vi "TAT_Start.vi"(8 "error In":errorcluster) -> (0 "error out":errorcluster)   [LabVIEW 2017]
uses:
  <vilib>/Utility/error.llb/DialogType.ctl
  Controls/Ass. Loop Control.ctl
  <vilib>/addons/database/Connection.llb/Conn ObjectReference.ctl
  2ffc4e95-467e-4723-8c12-a792954531b5.vi
  8539105e-fe5f-4c29-a376-e00596b22cdb.vi
  <vilib>/addons/database/Connection.llb/DB Tools Open Connec (Path).vi
  Global/Global 1.vi
  <vilib>/Instr/_visa.llb/VISA Configure Serial Port (Instr).vi
  <vilib>/addons/database/NI_Database_API.lvlib
  <vilib>/Utility/config.llb/NI_LVConfig.lvlib
panel:
  out "PREVIOUS BARCODE":string
  out "PACKAGED QUANTITY":string
  out "SCANNED QUANTITY":string
  out "PACKAGE STICKER":string
  out "PRN to Print":string
  out "CYCLE RESULT:-":bool caption="LEAK RESULT:-"
  out "CYCLE STATUS STATION 2":string caption="CYCLE STATUS 2:-"
  out "SERIAL NO.:- 2":dbl
  out "PY1B-D-EX:-":bool caption="LEAK RESULT:-"
  out "PYIB-MD-EX:-":bool caption="LEAK RESULT:-"
  out "RBC-M-H:-":bool caption="LEAK RESULT:-"
  out "PY1B-D:-":bool caption="LEAK RESULT:-"
  out "PYIB-MD:-":bool caption="LEAK RESULT:-"
  out "HOSE:-":bool caption="LEAK RESULT:-"
  out "DUAL:-":bool caption="LEAK RESULT:-"
  out "RBC-M-EX:-":bool caption="LEAK RESULT:-"
  out "CAP SEAL:-":bool caption="LEAK RESULT:-"
  in  "Model Selection:-":string(combo)
  out "CYCLE TIME:-":u32
  out "BARCODE STATION 2":string caption="QR CODE :-"
  out "CYCLE START:-":bool caption="LEAK RESULT:-"
  out "PREVIOUS BARCODE":string[](array[string])
  out "scanned":string
  out "Scanned Qty  2":string
  out "PROJECT :-":string
  out "PACKAGE Qty":string
  out "TORISHI CODE:-":string
  out "PART No.:-":string
  out "PLC STATUS:-":bool
  in  "Stop":bool
  out "QR STATION 1":string caption="QR CODE:-"
  out "RESULT STATION 1":bool caption="FINAL RESULT:-"
  out "USER:-":string
  out "PART NAME :-":string
  in  "ASS-Alarms":bool
  out "CYCLE STATUS STATION 1":string caption="CYCLE STATUS 1:-"
  out "DATE/TIME":string
  # "KAPSE SONS ROBOTICS\n& AUTOMATION"
  # "MODEL SELECTION:-"
  # "Nm"
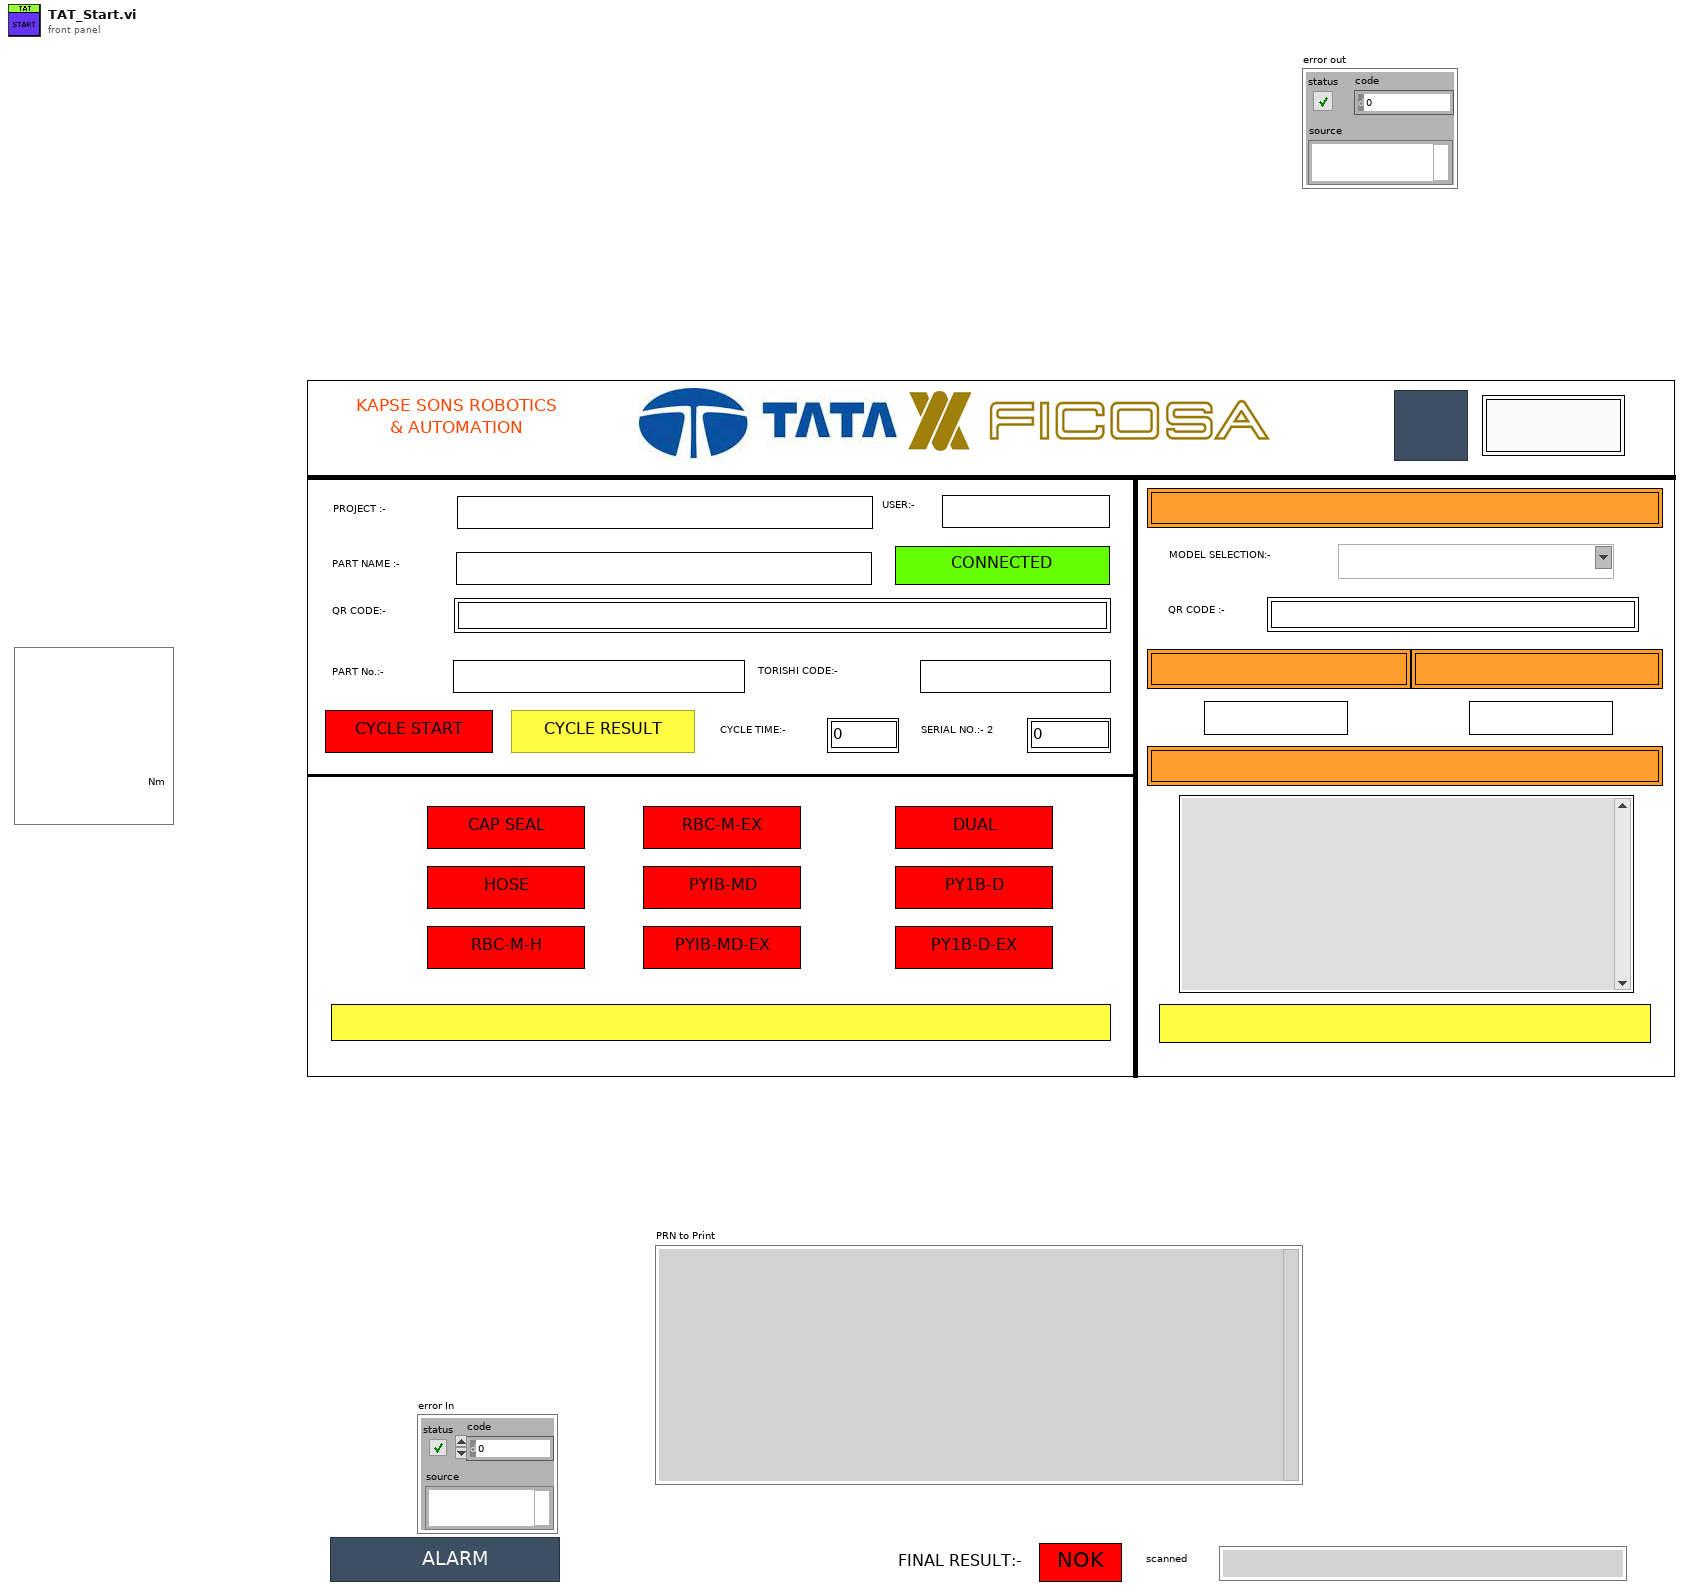
[diagram p1: front panel]
types:
  T1 = typedef "NI_Database_API.lvlib/Conn ObjectReference.ctl" = refnum<k1>
  T2 = cluster{"Varient number":u16, "Part name":string, "connection reference":T1, "Batch_Size":u16, "PART_NO":string, "TORISHI_CODE":string, "scanner com":refnum<visa-resource-name>, "Part Name List":string[], "Varient path":path, "Current Varient path":path, "Communication path":path, "Package path":path, "Part PRN path":path, "Station2 printer IP":string, "Station1 printer IP":string, "Current Serial Number":string, "Station1_QR":string, "Serial_Number":path, "PRIVIOUS code":string[], "Barcode station 2 to log Dn":string, "Barcode station 2 to log Up":string}
  T3 = cluster{"Varient number":u16, "Part name":string, "Barcode":string, "connection reference":T1, "Batch_Size":u16, "PART_NO":string, "TORISHI_CODE":string, "scanner com":refnum<visa-resource-name>, "Part Name List":string[], "Varient path":path, "Current Varient path":path, "Communication path":path, "Package path":path, "Part PRN path":path, "Station2 printer IP":string, "Station1 printer IP":string, "Current Serial Number":string, "Station1_QR":string, "Serial_Number":path, "PRIVIOUS code":string[], "Barcode station 2 to log":string}
  T4 = typedef "Ass. Loop Control.ctl" = enum16{"Package_Qty_Count", "GENERATE_QR_PRNT", "Cluster_update", "Waiting_for_scan", "barcode CHECK", "Int", "SaveReport ", "Barcode Print", "Start Cycle", "Wait", "Cycle End", "Stop"}
  T5 = typedef "DialogType.ctl" = u16
  T6 = enum32{"invalid app kind", "Development System", "Run Time System", "Student Edition", "Embedded LabVIEW", "Evaluation", "Custom"}
  T7 = typedef "NI_LVConfig.lvlib/Config Data RefNum.ctl" = refnum<k1>
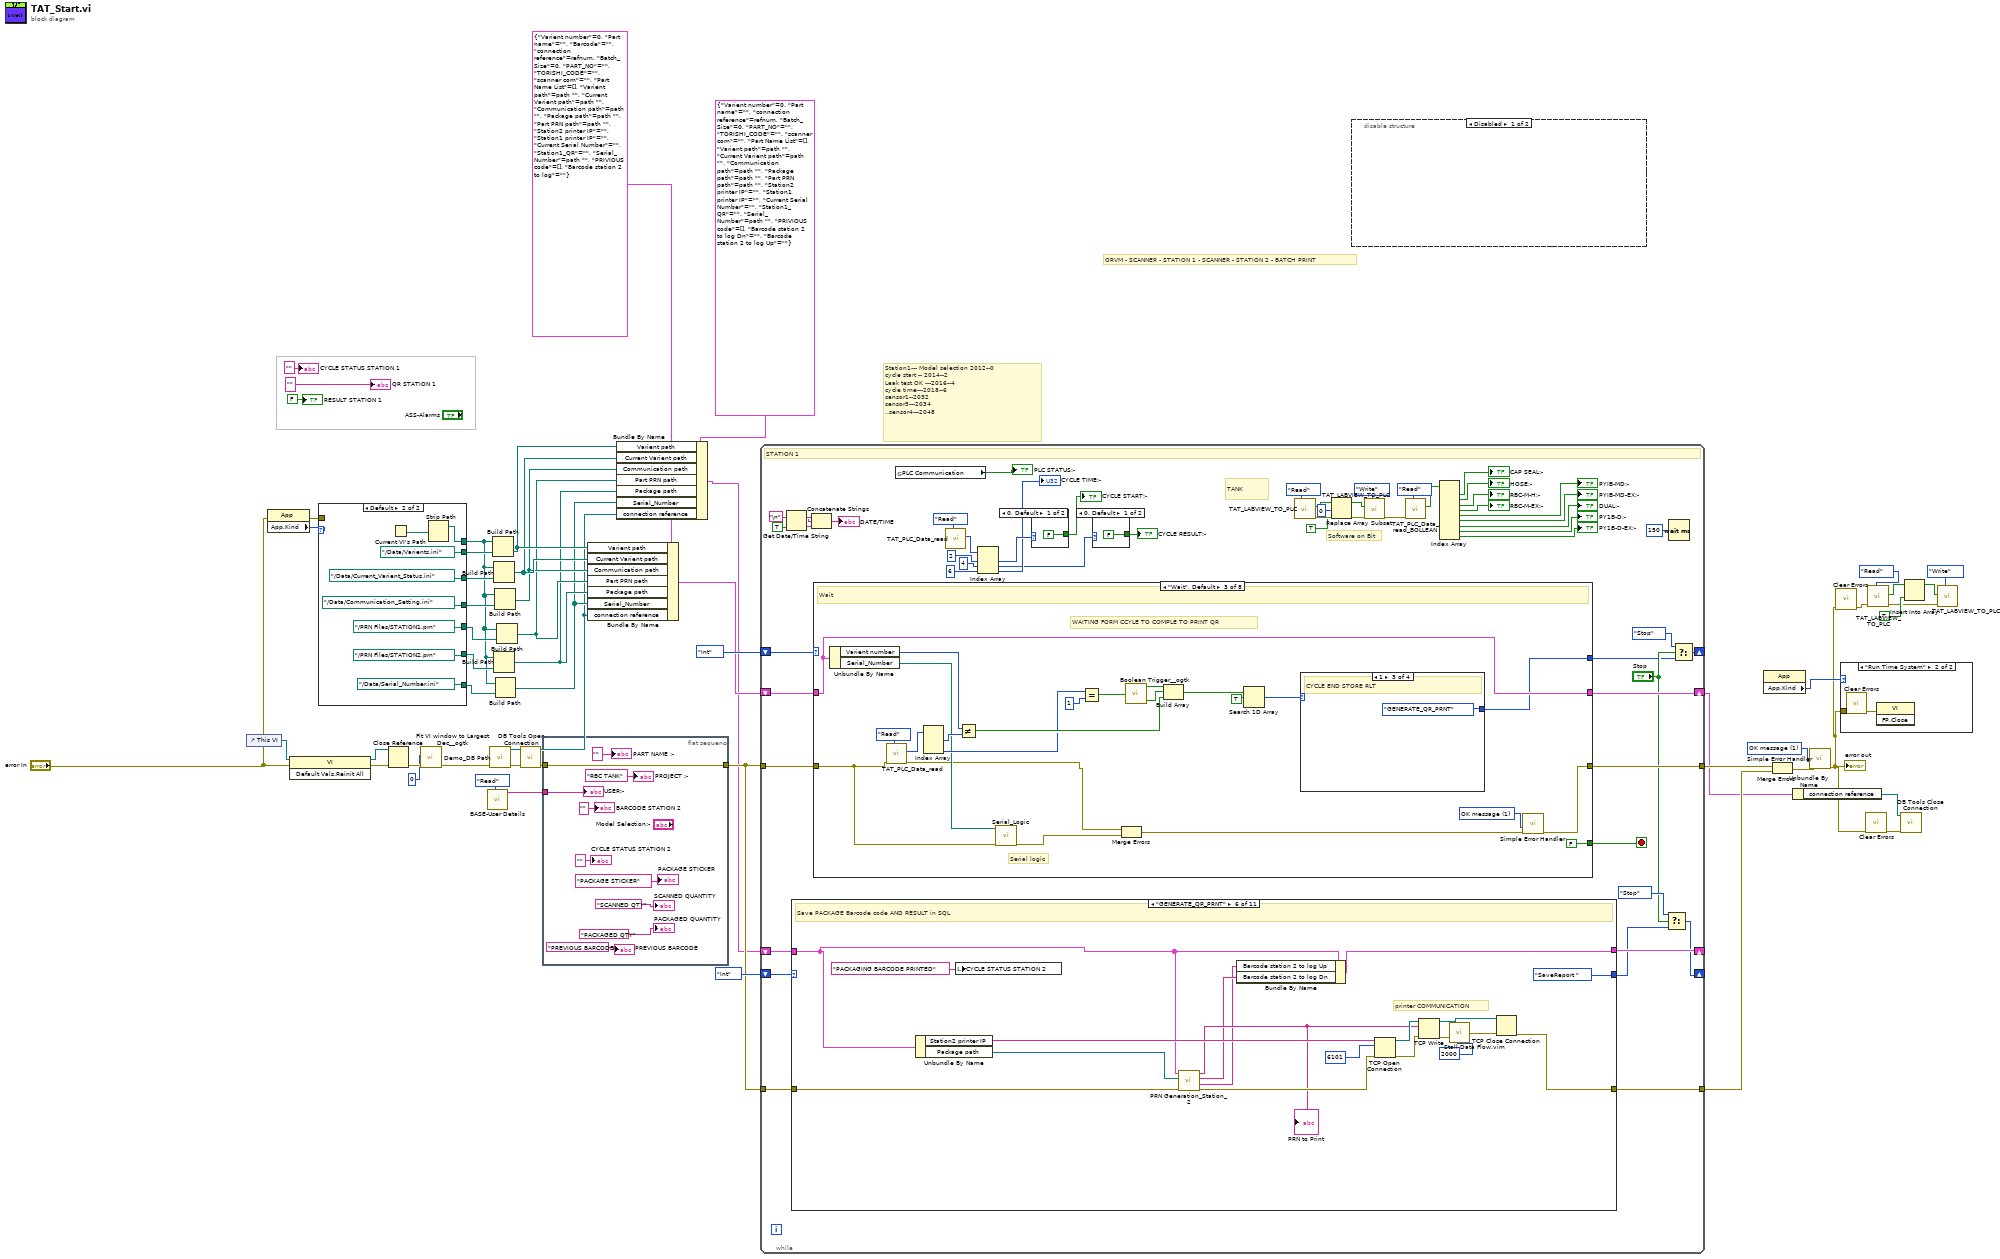
[diagram p0: block diagram]
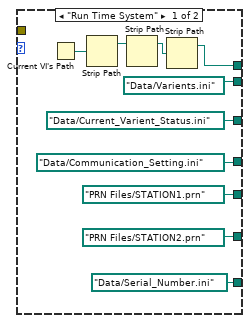
[diagram p2: hidden frame]
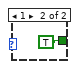
[diagram p5: hidden frame]
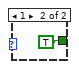
[diagram p6: hidden frame]
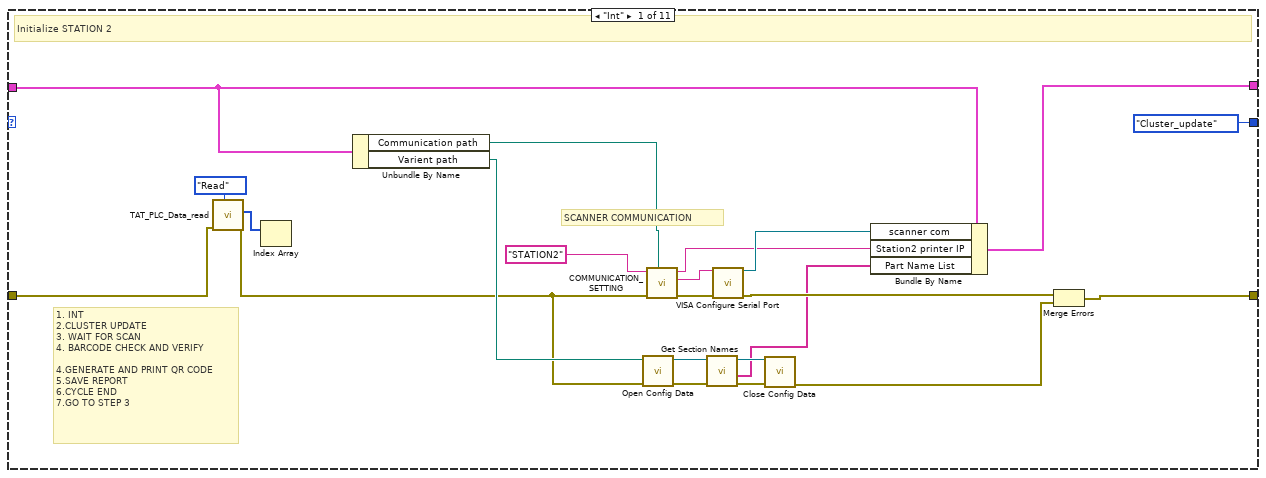
[diagram p7: hidden frame]
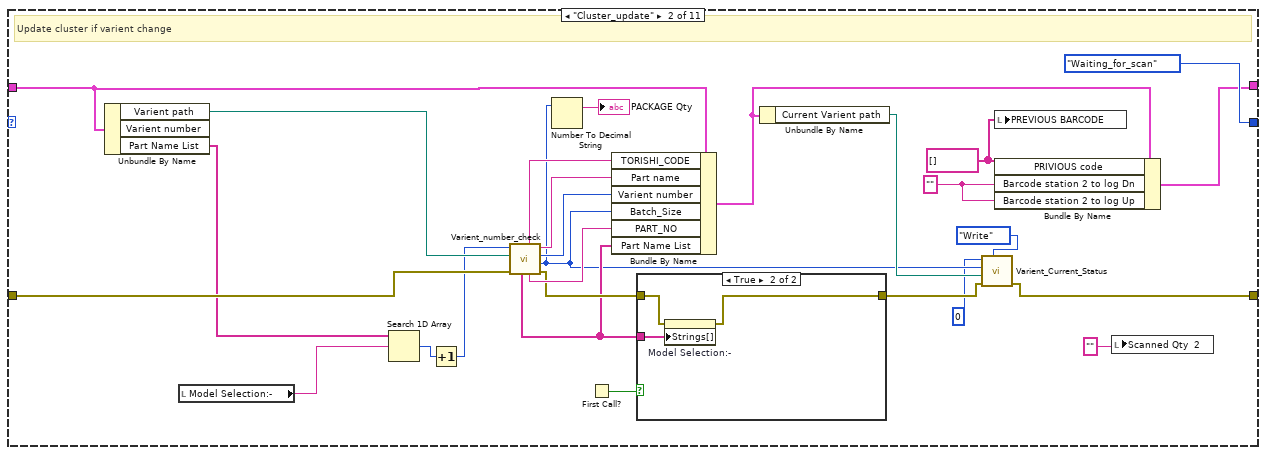
[diagram p8: hidden frame]
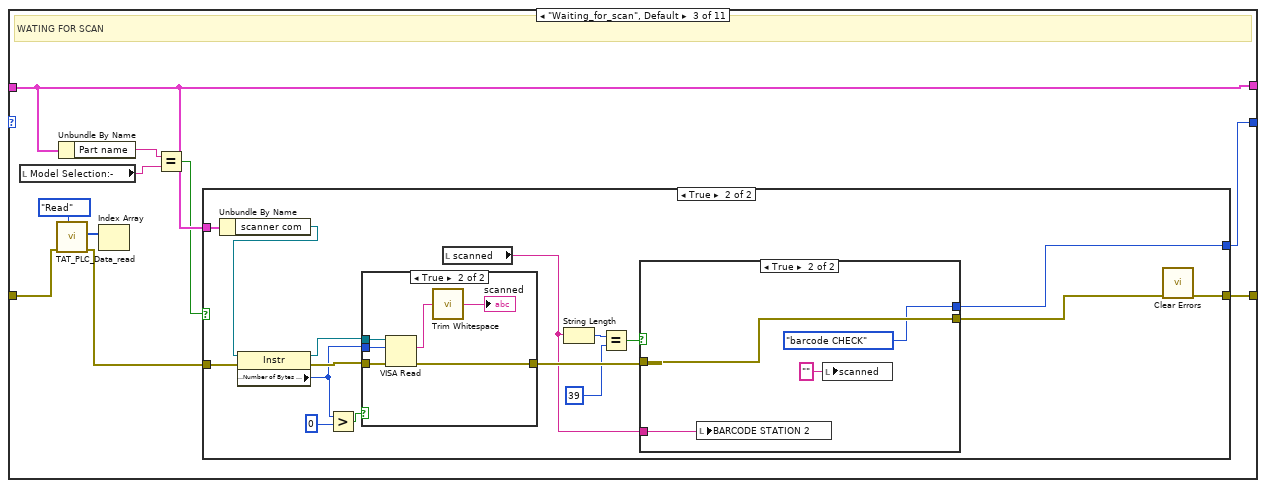
[diagram p10: hidden frame]
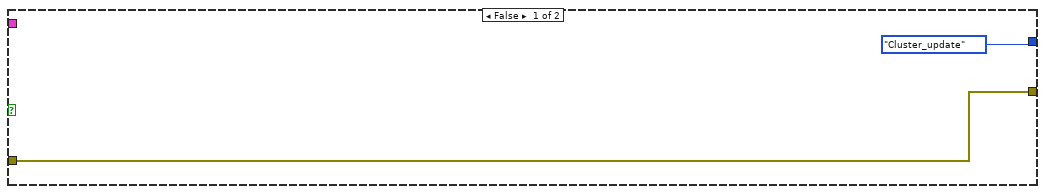
[diagram p11: hidden frame]
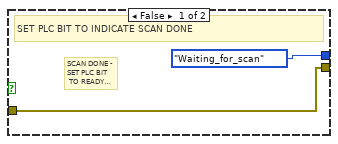
[diagram p13: hidden frame]
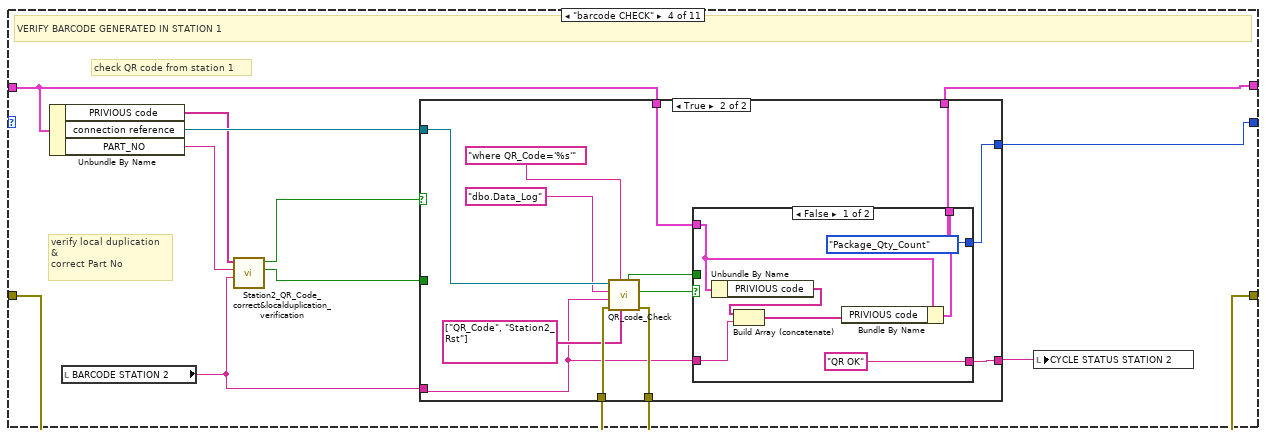
[diagram p14: hidden frame]
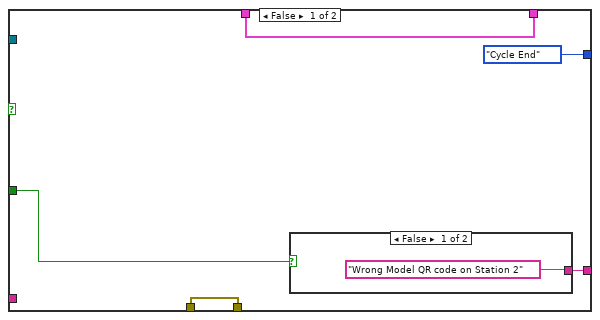
[diagram p15: hidden frame]
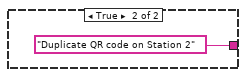
[diagram p16: hidden frame]
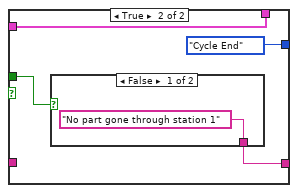
[diagram p17: hidden frame]
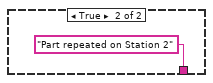
[diagram p18: hidden frame]
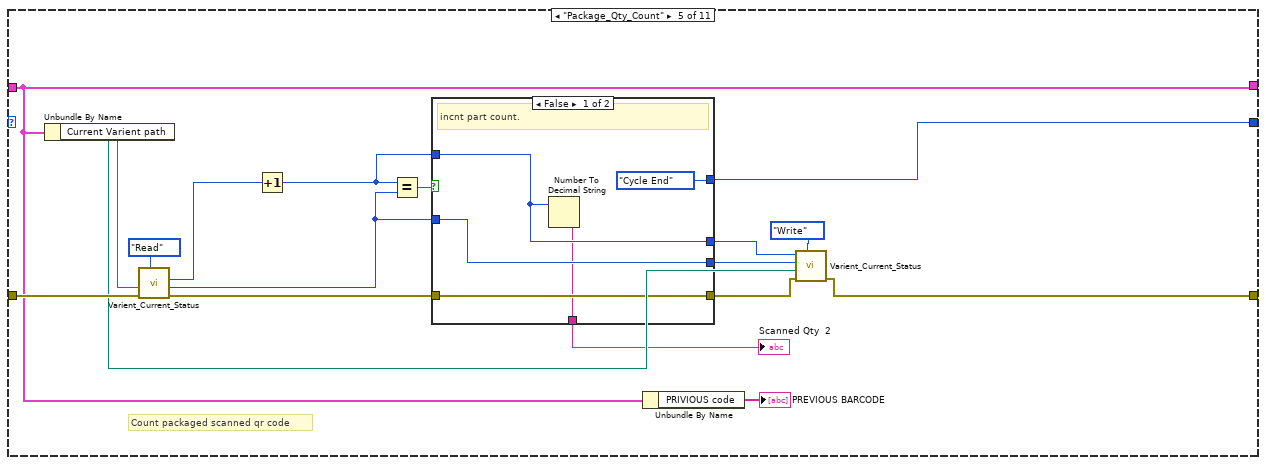
[diagram p19: hidden frame]
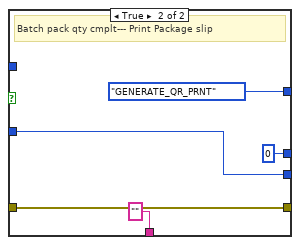
[diagram p20: hidden frame]
diagram:
  w42 = T5 1 items=["no dialog", "OK message", "continue or stop message", "OK message + warnings", "continue/stop + warnings"] ("type of dialog (OK msg:1)")
  # "Station1--- Model selection 2012--0\ncycle start -- 2014--2\nLeak test OK ---2016--4\ncycle time---2018--6\nsensor1--2032\nsensor3---2034\n..sensor4---2048"
  # "ORVM - SCANNER - STATION 1 - SCANNER - STATION 2 - BATCH PRINT"
  n1 = control-ref of="This VI"() -> (w54:refnum<vi>)
  n2 = property class="App"(error in="error In") -> (error out=w32:errorcluster, "App.Kind"=w37:T6)  [unwired: 1 in, 1 out]
  n3 = invoke class="VI" method="Default Vals.Reinit All"(reference=w54, error in="error In") -> (reference out=w52:refnum<vi>, error out=w53:errorcluster)  [unwired: 1 in, 1 out]
  n4 = case shown="Default" w37 {
    tunnel: [path "Data/Varients.ini" ("path") path "../Data/Varients.ini" ("path")] -> w36
    tunnel: [w60 w70] -> w27
    tunnel: [path "Data/Current_Varient_Status.ini" ("path") path "../Data/Current_Varient_Status.ini" ("path")] -> w35
    tunnel: [path "Data/Communication_Setting.ini" ("path") path "../Data/Communication_Setting.ini" ("path")] -> w34
    tunnel: [path "PRN Files/STATION2.prn" ("path") path "../PRN Files/STATION2.prn" ("path")] -> w33
    tunnel: w32 -> [_ _]
    tunnel: [path "PRN Files/STATION1.prn" ("path") path "../PRN Files/STATION1.prn" ("path")] -> w30
    tunnel: [path "Data/Serial_Number.ini" ("path") path "../Data/Serial_Number.ini" ("path")] -> w26
    frame "Run Time System" {
      n5 = Current VI's Path() -> (path=w63:path)
      n6 = Strip Path(path=w63) -> (stripped path=w62:path)  [unwired: 1 out]
      n7 = Strip Path(path=w62) -> (stripped path=w61:path)  [unwired: 1 out]
      n8 = Strip Path(path=w61) -> (stripped path=w60:path)  [unwired: 1 out]
    }
    frame Default {
      n9 = Current VI's Path() -> (path=w71:path)
      n10 = Strip Path(path=w71) -> (stripped path=w70:path)  [unwired: 1 out]
    }
  }
  n11 = Close Reference(reference=w52, error in (no error)=w53) -> (error out=w51:errorcluster)
  n12 = call <userlib>:"Fit VI window to Largest Dec__ogtk.vi"("error in (no error)"=w51, "border spacing (2 px)"=0) -> ("error out"=w16:errorcluster)  [unwired: 4 in, 1 out]
  n13 = call "BASE-User Details.vi"("Enum"=enum16{"Read", "Write"}."Read") -> ("User Name Out"=w43:string)  [unwired: 9 in, 1 out]
  n14 = call "Demo_DB Path.vi"("error in"=w16) -> ("error out"=w18:errorcluster, "DB Path"=w17:path)  [unwired: 9 in]
  n15 = Build Path(base path=w27, name or relative path=w36) -> (appended path=w10:path)
  n16 = Build Path(base path=w27, name or relative path=w35) -> (appended path=w9:path)
  n17 = Build Path(base path=w27, name or relative path=w33) -> (appended path=w6:path)
  n18 = Build Path(base path=w27, name or relative path=w34) -> (appended path=w8:path)
  n19 = Build Path(base path=w27, name or relative path=w26) -> (appended path=w5:path)
  n20 = Build Path(base path=w27, name or relative path=w30) -> (appended path=w7:path)
  n21 = call-poly <vilib>:"DB Tools Open Connection.vi"("error in (no error)"=w18, "connection information"=w17) -> ("error out"=w15:errorcluster, "connection reference"=w4:T1)  [unwired: 6 in]
  n22 = flat-sequence {
    tunnel: [w82] -> w40
    tunnel: w15 -> [w82]
    tunnel: w43 -> [w80]
    frame #0 {
      "USER:-" <- w80
      "PART NAME :-" <- ""
      "PROJECT :-" <- "RBC TANK" ("PROJECT")
      "BARCODE STATION 2" <- "" ("BARCODE STATION 2")
      "CYCLE STATUS STATION 2" <- "" ("CYCLE STATUS STATION 2")
      "PACKAGE STICKER" <- "PACKAGE STICKER" ("PACKAGE STICKER")
      "SCANNED QUANTITY" <- "SCANNED QTY" ("PACKAGE STICKER")
      "PACKAGED QUANTITY" <- "PACKAGED QTY" ("PACKAGE STICKER")
      "PREVIOUS BARCODE" <- "PREVIOUS BARCODE" ("PACKAGE STICKER")
    }
  }
  n23 = Bundle By Name(cluster=T3 {"Varient number"=0, "Part name"="", "Barcode"="", "connection reference"=refnum, "Batch_Size"=0, "PART_NO"="", "TORISHI_CODE"="", "scanner com"="", "Part Name List"=[], "Varient path"=path "", "Current Varient path"=path "", "Communication path"=path "", "Package path"=path "", "Part PRN path"=path "", "Station2 printer IP"="", "Station1 printer IP"="", "Current Serial Number"="", "Station1_QR"="", "Serial_Number"=path "", "PRIVIOUS code"=[], "Barcode station 2 to log"=""}, "Varient path"=w10, "Current Varient path"=w9, "Communication path"=w8, "Part PRN path"=w7, "Package path"=w6, "Serial_Number"=w5, "connection reference"=w4) -> (w28:T3)
  n24 = Bundle By Name(cluster=T2 {"Varient number"=0, "Part name"="", "connection reference"=refnum, "Batch_Size"=0, "PART_NO"="", "TORISHI_CODE"="", "scanner com"="", "Part Name List"=[], "Varient path"=path "", "Current Varient path"=path "", "Communication path"=path "", "Package path"=path "", "Part PRN path"=path "", "Station2 printer IP"="", "Station1 printer IP"="", "Current Serial Number"="", "Station1_QR"="", "Serial_Number"=path "", "PRIVIOUS code"=[], "Barcode station 2 to log Dn"="", "Barcode station 2 to log Up"=""}, "Varient path"=w10, "Current Varient path"=w9, "Communication path"=w8, "Part PRN path"=w7, "Package path"=w6, "Serial_Number"=w5, "connection reference"=w4) -> (w2:T2)
  n25 = while {
    tunnel: w40 -> [w131]
    shift-right: [w130] -> _
    shift-left: Ass._Loop_Control."Int" ("Enum") -> [w136]
    shift-right: [w134] -> w11
    shift-left: w28 -> [w133]
    tunnel: [w132] -> w47
    shift-right: [w116] -> _
    shift-left: Ass._Loop_Control."Int" ("Enum") -> [w122]
    tunnel: w40 -> [w121]
    shift-right: [w119] -> _
    shift-left: w2 -> [w120]
    tunnel: [w118] -> w39
    stop <- w123 stop-if-true
    # "Software on Bit"
    # "TANK"
    # "STATION 1"
    n26 = Get Date/Time String(want seconds? (F)=TRUE) -> (date string=w127:string, time string=w126:string)  [unwired: 2 in]
    n27 = case shown="\"GENERATE_QR_PRNT\"" w122 {
      tunnel: [Ass._Loop_Control."Cluster_update" ("Enum") Ass._Loop_Control."Waiting_for_scan" ("Enum") w202 w239 w284 Ass._Loop_Control."SaveReport " ("Enum") Ass._Loop_Control."Cycle End" ("Enum") Ass._Loop_Control."Waiting_for_scan" ("Enum") Ass._Loop_Control."Stop" ("Enum") w348 Ass._Loop_Control."Wait" ("Enum")] -> w115
      tunnel: [w159 w165 w197 w245 w283 w309 w330 w333 w338 w342 w358] -> w119
      tunnel: [w147 w171 w203 w243 w290 w316 w329 w334 w339 w344 w359] -> w118
      tunnel: w121 -> [w142 w188 w199 w244 w296 w314 w331 w334 w336 _ w359]
      tunnel: w120 -> [w155 w181 w197 w246 w283 w310 w328 w333 w338 w342 w358]
      frame "Int" {
        # "1. INT\n2.CLUSTER UPDATE\n3. WAIT FOR SCAN\n4. BARCODE CHECK AND VERIFY\n\n4.GENERATE AND PRINT QR CODE\n5.SAVE REPORT\n6.CYCLE END\n7.GO TO STEP 3"
        # "SCANNER COMMUNICATION"
        # "Initialize STATION 2"
        n28 = call "TAT_PLC_Data_read.vi"("Enum"=enum16{"Read", "Write"}."Read", "error in (no error)"=w142) -> ("error out"=w141:errorcluster, "Array 2"=w144:u16[])  [unwired: 8 in]
        n29 = Index Array(array=w144) -> ()  [unwired: 1 in, 1 out]
        n30 = Unbundle By Name(w155) -> ("Communication path"=w154:path, "Varient path"=w145:path)
        n31 = call <vilib>:"Open Config Data.vi"("error in (no error)"=w141, "configuration file path"=w145) -> ("error out"=w152:errorcluster, "refnum"=w153:T7)  [unwired: 7 in, 1 out]
        n32 = call "COMMUNICATION_SETTING.vi"("communication path"=w154, "error in"=w141, "STATION"="STATION2") -> ("error out"=w161:errorcluster, "SCAN_COM"=w157:string, "PRINT_COM"=w156:string)  [unwired: 6 in]
        n33 = call <vilib>:"Get Section Names.vi"("error in (no error)"=w152, "refnum"=w153) -> ("error out"=w151:errorcluster, "section names"=w146:string[], "refnum out"=w150:T7)  [unwired: 7 in]
        n34 = call-poly "VISA Configure Serial Port"("VISA resource name"=w157, "error in (no error)"=w161) -> ("VISA resource name out"=w158:refnum<visa-resource-name>, "error out"=w148:errorcluster)  [unwired: 12 in]
        n35 = call <vilib>:"Close Config Data.vi"("error in (no error)"=w151, "refnum"=w150) -> ("error out"=w149:errorcluster)  [unwired: 8 in, 1 out]
        n36 = Bundle By Name(cluster=w155, "scanner com"=w158, "Station2 printer IP"=w156, "Part Name List"=w146) -> (w159:T2)
        n37 = Merge Errors(w148, w149) -> (w147:errorcluster)
      }
      frame "Cluster_update" {
        w163 = "" ("Barcode station 2 to log")
        w164 = string[] [] ("PREVIOUS Code")
        # "Update cluster if varient change"
        n38 = Unbundle By Name(w181) -> ("Varient path"=w187:path, "Part Name List"=w178:string[])  [unwired: 1 out]
        n39 = local read "Model Selection:-"() -> (w176:string)
        n40 = Search 1D Array(1D array=w178, element=w176) -> (index of element=w180:i32)  [unwired: 1 in]
        n41 = Increment(x=w180) -> (x+1=w177:i32)
        n42 = call "Varient_number_check.vi"("error in"=w188, "Varient path"=w187, "Varient No."=w177) -> ("error out"=w182:errorcluster, "Batch Size"=w169:i32, "Varient Number"=w174:i32, "Part Name"=w185:string, "PART_NO"=w184:string, "TORISHI_CODE"=w186:string, "MODEL LIST"=w179:string[])  [unwired: 2 in]
        n43 = Number To Decimal String(number=w169) -> (decimal integer string=→"PACKAGE Qty":string)  [unwired: 1 in]
        n44 = First Call?() -> (First Call?: T/F=w175:bool)
        n45 = Bundle By Name(cluster=w181, "TORISHI_CODE"=w186, "Part name"=w185, "Varient number"=w174, "Batch_Size"=w169, "PART_NO"=w184, "Part Name List"=w179) -> (w166:T2)
        n46 = case shown="True" w175 {
          tunnel: w182 -> [w190 w193]
          tunnel: [w190 w192] -> w172
          tunnel: w179 -> [_ w191]
          frame False {
          }
          frame True {
            n47 = property on="Model Selection:-" class="CmbBox"(error in=w193, "Strings[]"=w191) -> (error out=w192:errorcluster)  [unwired: 1 in, 1 out]
          }
        }
        n48 = Unbundle By Name(w166) -> ("Current Varient path"=w170:path)
        n49 = call "Varient_Current_Status.vi"("Enum"=enum16{"Write", "Read"}."Write", "error in"=w172, "Current Varient Status"=w170, "Batch Size"=w169, "Varient count"=0) -> ("error out"=w171:errorcluster)  [unwired: 4 in, 2 out]
        n50 = local write "PREVIOUS BARCODE"(w164) -> ()
        n51 = Bundle By Name(cluster=w166, "PRIVIOUS code"=w164, "Barcode station 2 to log Dn"=w163, "Barcode station 2 to log Up"=w163) -> (w165:T2)
        n52 = local write "Scanned Qty  2"("") -> ()
      }
      frame "Waiting_for_scan", Default {
        # "WATING FOR SCAN"
        n53 = local read "Model Selection:-"() -> (w195:string)
        n54 = call "TAT_PLC_Data_read.vi"("Enum"=enum16{"Read", "Write"}."Read", "error in (no error)"=w199) -> ("error out"=w198:errorcluster, "Array 2"=w201:u16[])  [unwired: 8 in]
        n55 = Unbundle By Name(w197) -> ("Part name"=w196:string)
        n56 = Index Array(array=w201) -> ()  [unwired: 1 in, 1 out]
        n57 = Equal?(x=w196, y=w195) -> (x = y?=w194:bool)
        n58 = case shown="True" w194 {
          tunnel: [w205 w221] -> w203
          tunnel: [Ass._Loop_Control."Cluster_update" ("Enum") w216] -> w202
          tunnel: w198 -> [w205 w215]
          tunnel: w197 -> [_ w214]
          frame False {
          }
          frame True {
            n59 = Unbundle By Name(w214) -> ("scanner com"=w213:refnum<visa-resource-name>)
            n60 = property class="Instr"(reference=w213, error in=w215) -> (reference out=w220:refnum<visa-resource-name>, error out=w219:errorcluster, "Serial Settings:Number of Bytes at Serial Port"=w206:u32)
            n61 = Greater?(x=w206, y=u32 0) -> (0:w207:bool)
            n62 = case shown="True" w207 {
              tunnel: w220 -> [_ w228]
              tunnel: w219 -> [w222 w227]
              tunnel: w206 -> [_ w226]
              tunnel: [w222 w225] -> w218
              frame False {
              }
              frame True {
                n63 = VISA Read(VISA resource name=w228, byte count=w226, error in (no error)=w227) -> (read buffer=w224:string, error out=w225:errorcluster)  [unwired: 2 out]
                n64 = call <vilib>:"Trim Whitespace.vi"("string"=w224) -> ("trimmed string"=→"scanned":string)  [unwired: 1 in]
              }
            }
            n65 = local read "scanned"() -> (w210:string)
            n66 = String Length(string=w210) -> (length=w212:i32)
            n67 = Equal?(x=w212, y=39) -> (x = y?=w209:bool)
            n68 = case shown="True" w209 {
              tunnel: w218 -> [w230 w234]
              tunnel: [w230 w234] -> w217
              tunnel: w210 -> [_ w231]
              tunnel: [Ass._Loop_Control."Waiting_for_scan" ("Enum") Ass._Loop_Control."barcode CHECK" ("Enum")] -> w216
              frame False {
                # "SCAN DONE - SET PLC BIT\n TO READY CYCLE"
                # "SET PLC BIT TO INDICATE SCAN DONE"
              }
              frame True {
                n69 = local write "BARCODE STATION 2"(w231) -> ()
                n70 = local write "scanned"("" ("scanned")) -> ()
              }
            }
            n71 = call <vilib>:"Clear Errors.vi"("error in (no error)"=w217) -> ("error out"=w221:errorcluster)  [unwired: 5 in, 1 out]
          }
        }
      }
      frame "barcode CHECK" {
        # "verify local duplication\n&\ncorrect Part No"
        # "check QR code from station 1"
        # "VERIFY BARCODE GENERATED IN STATION 1"
        n72 = Unbundle By Name(w246) -> ("PRIVIOUS code"=w238:string[], "connection reference"=w242:T1, "PART_NO"=w241:string)
        n73 = local read "BARCODE STATION 2"() -> (w237:string)
        n74 = call "Station2_QR_Code_correct&localduplication_verification.vi"("BARCODE STATION in"=w237, "PART_NO"=w241, "PRIVIOUS code"=w238) -> ("Correct part no True"=w235:bool, "Correct part no & No duplication TRUE"=w236:bool)  [unwired: 7 in]
        n75 = case shown="True" w236 {
          tunnel: w246 -> [w251 w266]
          tunnel: [w251 w265] -> w245
          tunnel: w244 -> [w250 w264]
          tunnel: [w250 w263] -> w243
          tunnel: w242 -> [_ w262]
          tunnel: w237 -> [_ w257]
          tunnel: [w249 w259] -> w240
          tunnel: [Ass._Loop_Control."Cycle End" ("Enum") w258] -> w239
          tunnel: w235 -> [w247 _]
          frame False {
            n76 = case shown="False" w247 {
              tunnel: ["Wrong Model QR code on Station 2" ("Cycle Status") "Duplicate QR code on Station 2" ("Cycle Status")] -> w249
              frame False {
              }
              frame True {
              }
            }
          }
          frame True {
            n77 = call "QR_code_Check.vi"("Columns"=string[] ["QR_Code", "Station2_Rst"] ("columns 2"), "format string"="where QR_Code='%s'", "error in (no error)"=w264, "replace %s"=w257, "table"="dbo.Data_Log", "Refnum in"=w262) -> ("error out"=w263:errorcluster, "FALSE healty"=w255:bool, "TRUE Duplication on Station 2"=w254:bool)  [unwired: 2 out]
            n78 = case shown="False" w255 {
              tunnel: ["QR OK" ("Cycle Status") w277] -> w259
              tunnel: w266 -> [w270 w276]
              tunnel: [w272 w276] -> w265
              tunnel: [Ass._Loop_Control."Package_Qty_Count" ("Enum") Ass._Loop_Control."Cycle End" ("Enum")] -> w258
              tunnel: w257 -> [w267 _]
              tunnel: w254 -> [_ w274]
              frame False {
                n79 = Unbundle By Name(w270) -> ("PRIVIOUS code"=w269:string[])
                n80 = Build Array (concatenate)(w269, w267) -> (w268:string[])
                n81 = Bundle By Name(cluster=w270, "PRIVIOUS code"=w268) -> (w272:T2)
              }
              frame True {
                n82 = case shown="False" w274 {
                  tunnel: ["No part gone through station 1" ("Cycle Status") "Part repeated on Station 2" ("Cycle Status")] -> w277
                  frame False {
                  }
                  frame True {
                  }
                }
              }
            }
          }
        }
        n83 = local write "CYCLE STATUS STATION 2"(w240) -> ()
      }
      frame "Package_Qty_Count" {
        # "Count packaged scanned qr code"
        n84 = Unbundle By Name(w283) -> ("Current Varient path"=w282:path)
        n85 = call "Varient_Current_Status.vi"("Enum"=enum16{"Write", "Read"}."Read", "error in"=w296, "Current Varient Status"=w282) -> ("error out"=w294:errorcluster, "Batch Size"=w287:i32, "Varient Count"=w293:i32)  [unwired: 6 in]
        n86 = Increment(x=w293) -> (x+1=w288:i32)
        n87 = Equal?(x=w288, y=w287) -> (x = y?=w292:bool)
        n88 = case shown="False" w292 {
          tunnel: [w301 w306] -> w289
          tunnel: w294 -> [w301 w306]
          tunnel: w288 -> [w298 _]
          tunnel: w287 -> [w300 w305]
          tunnel: [w300 w305] -> w286
          tunnel: [w298 0] -> w285
          tunnel: [Ass._Loop_Control."Cycle End" ("Enum") Ass._Loop_Control."GENERATE_QR_PRNT" ("Enum")] -> w284
          tunnel: [w297 "" ("String")] -> w281
          frame False {
            # "incnt part count."
            n89 = Number To Decimal String(number=w298) -> (decimal integer string=w297:string)  [unwired: 1 in]
          }
          frame True {
            # "Batch pack qty cmplt--- Print Package slip"
          }
        }
        "Scanned Qty  2" <- w281
        n90 = Unbundle By Name(w283) -> ("PRIVIOUS code"=→"PREVIOUS BARCODE":string[])
        n91 = call "Varient_Current_Status.vi"("Enum"=enum16{"Write", "Read"}."Write", "error in"=w289, "Current Varient Status"=w282, "Batch Size"=w286, "Varient count"=w285) -> ("error out"=w290:errorcluster)  [unwired: 4 in, 2 out]
      }
      frame "GENERATE_QR_PRNT" {
        # "printer COMMUNICATION"
        # "Save PACKAGE Barcode code AND RESULT in SQL"
        n92 = Unbundle By Name(w310) -> ("Station2 printer IP"=w315:string, "Package path"=w312:path)
        n93 = local write "CYCLE STATUS STATION 2"("PACKAGING BARCODE PRINTED" ("Cycle Status")) -> ()
        n94 = call "PRN Generation_Station_2.vi"("error in (no error)"=w314, "PRN path"=w312, "Cluster"=w310) -> ("error out"=w313:errorcluster, "Barcode Station 2 Up"=w307:string, "Barcode station 2 Dn"=w308:string, "PRN to Print"=w311:string)  [unwired: 5 in]
        "PRN to Print" <- w311
        n95 = Bundle By Name(cluster=w310, "Barcode station 2 to log Up"=w307, "Barcode station 2 to log Dn"=w308) -> (w309:T2)
        n96 = TCP Open Connection(address=w315, remote port or service name=u16 6101, error in (no error)=w313) -> (connection ID=w321:refnum<k5>, error out=w322:errorcluster)  [unwired: 2 in]
        n97 = TCP Write(connection ID=w321, data in=w311, error in (no error)=w322) -> (connection ID out=w319:refnum<k5>, error out=w323:errorcluster)  [unwired: 1 in, 1 out]
        n98 = call "Stall Data Flow.vim"("value in"=w323, "milliseconds to wait"=u32 2000) -> ("value out"=w320:errorcluster)  [unwired: 1 out]
        n99 = TCP Close Connection(connection ID=w319, error in (no error)=w320) -> (error out=w316:errorcluster)  [unwired: 1 in, 1 out]
      }
      frame "SaveReport " {
        w326 = "" ("Barcode station 2 to log")
        w327 = string[] [] ("PREVIOUS Code")
        # "Save Barcode code AND RESULT in SQL"
        n100 = call "Station2_Data_Log.vi"("error in (no error)"=w331, "Cluster"=w328) -> ("error out"=w329:errorcluster)  [unwired: 9 in]
        n101 = Bundle By Name(cluster=w328, "PRIVIOUS code"=w327, "Barcode station 2 to log Dn"=w326, "PRIVIOUS code"=w327, "Barcode station 2 to log Up"=w326) -> (w330:T2)
        n102 = local write "PREVIOUS BARCODE"(w327) -> ()
      }
      frame "Cycle End" {
      }
      frame "Stop" {
        n103 = local write "CYCLE STATUS STATION 2"("STATION STOP" ("Cycle Status")) -> ()
        n104 = Unbundle By Name(w338) -> ("scanner com"=w337:refnum<visa-resource-name>)
        n105 = VISA Close(VISA resource name=w337, error in (no error)=w336) -> (error out=w339:errorcluster)
      }
      frame "Wait" {
        (unwired) FALSE
        # "Wait-- NOT USED"
        n106 = disable-structure shown="Disabled" {
          frame Disabled {
            # "PLC INT AND BITS"
            n107 = call "TAT_PLC_Data_read.vi"("Enum"=enum16{"Read", "Write"}."Read") -> ()  [unwired: 9 in, 2 out]
          }
          frame Enabled {
          }
        }
        n108 = call "TAT_PLC_Data_read_BOLLEAN.vi"("Enum"=enum16{"Read", "Write"}."Read") -> ("error out"=w344:errorcluster, "Array 2"=w345:bool[])  [unwired: 9 in]
        n109 = Index Array(array=w345, index=2) -> (element=w346:bool)
        n110 = call <userlib>:"Boolean Trigger__ogtk.vi"("Boolean Input"=w346) -> ("Rising Edge"=w352:bool, "Falling Edge"=w350:bool)  [unwired: 1 in]
        n111 = Build Array(w352, w350) -> (w351:bool[])
        n112 = Search 1D Array(1D array=w351, element=TRUE ("Boolean Input")) -> (index of element=w349:i32)  [unwired: 1 in]
        n113 = case shown="-1, Default" w349 {
          tunnel: [Ass._Loop_Control."Wait" ("Enum") Ass._Loop_Control."Start Cycle" ("Enum") Ass._Loop_Control."SaveReport " ("Enum")] -> w348
          frame -1, Default {
          }
          frame 0 {
            # "CYCYLE START BIT"
          }
          frame 1 {
            # "CYCLE END STORE RLT"
          }
        }
      }
      frame "Start Cycle" {
        n114 = local write "CYCLE STATUS STATION 1"("Cycle started" ("Cycle Status")) -> ()
      }
    }
    n115 = Concatenate Strings(w127, "\n", w126) -> (→"DATE/TIME":string)
    n116 = case shown="\"Wait\", Default" w136 {
      tunnel: [Ass._Loop_Control."Cluster_update" ("Enum") Ass._Loop_Control."Wait" ("Enum") w407 Ass._Loop_Control."Wait" ("Enum") w434 Ass._Loop_Control."Cycle End" ("Enum") Ass._Loop_Control."Wait" ("Enum") Ass._Loop_Control."Stop" ("Enum")] -> w113
      tunnel: [w369 w377 w409 w426 w432 w480 w489 w492] -> w134
      tunnel: w133 -> [w363 w376 w409 w426 w433 w480 w489 w492]
      tunnel: [_ _ FALSE _ _ _ _ TRUE] -> w123
      tunnel: [w367 w379 w396 w423 w427 w472 w488 w490] -> w132
      tunnel: w131 -> [w362 w384 w402 w423 w438 w485 w488 w490]
      frame "Int" {
        w368 = T5 1 items=["no dialog", "OK message", "continue or stop message", "OK message + warnings", "continue/stop + warnings"] ("type of dialog (OK msg:1)")
        # "1. INT\n2.CLUSTER UPDATE\n3. WAIT\n4.GENERATE AND PRINT QR CODE\n5.SAVE REPORT\n6.CYCLE END\n7.GO TO STEP 3"
        # "Initialize"
        n117 = Unbundle By Name(w363) -> ("Communication path"=w365:path)
        n118 = local write "CYCLE STATUS STATION 1"("WAIT FOR CYCLE START" ("Cycle Status")) -> ()
        n119 = call "COMMUNICATION_SETTING.vi"("communication path"=w365, "error in"=w362, "STATION"="STATION1") -> ("error out"=w366:errorcluster, "PRINT_COM"=w364:string)  [unwired: 6 in, 1 out]
        n120 = Bundle By Name(cluster=w363, "Station1 printer IP"=w364) -> (w369:T3)
        n121 = call <vilib>:"Simple Error Handler.vi"("type of dialog (OK msg:1)"=w368, "error in (no error)"=w366) -> ("error out"=w367:errorcluster)  [unwired: 3 in, 4 out]
      }
      frame "Cluster_update" {
        # "PART NAME\nPART No.\nPACKAGE QUANTITY\nTORISHI CODE"
        # "PART NAME---\nVARIENT NAME"
        # "Update cluster if varient change"
        n122 = Unbundle By Name(w376) -> ("Varient path"=w375:path)
        n123 = call "TAT_PLC_Data_read.vi"("Enum"=enum16{"Read", "Write"}."Read", "error in (no error)"=w384) -> ("error out"=w381:errorcluster, "Array 2"=w386:u16[])  [unwired: 8 in]
        n124 = Index Array(array=w386) -> (element=w374:u16)  [unwired: 1 in]
        n125 = call "Varient_number_check.vi"("error in"=w381, "Varient path"=w375, "Varient No."=w374) -> ("error out"=w380:errorcluster, "Batch Size"=w378:i32, "Part Name"=w383:string, "PART_NO"=w382:string, "TORISHI_CODE"=w373:string)  [unwired: 2 in, 2 out]
        "PART No.:-" <- w382
        "TORISHI CODE:-" <- w373
        n126 = Bundle By Name(cluster=w376, "Part name"=w383, "Varient number"=w374, "Batch_Size"=w378, "PART_NO"=w382, "TORISHI_CODE"=w373) -> (w377:T3)
        n127 = local write "PART NAME :-"(w383) -> ()
        n128 = disable-structure shown="Disabled" {
          disable-tunnel: w380 -> [w393 w395]
          disable-tunnel: [w392 w395] -> w379
          disable-tunnel: w378 -> [w391 _]
          disable-tunnel: w377 -> [w389 _]
          frame Disabled {
            n129 = Unbundle By Name(w389) -> ("Current Varient path"=w388:path)
            n130 = call "Varient_Current_Status.vi"("Enum"=enum16{"Write", "Read"}."Write", "error in"=w393, "Current Varient Status"=w388, "Batch Size"=w391, "Varient count"=0) -> ("error out"=w392:errorcluster)  [unwired: 4 in, 2 out]
          }
          frame Enabled {
          }
        }
      }
      frame "Wait", Default {
        w398 = T5 1 items=["no dialog", "OK message", "continue or stop message", "OK message + warnings", "continue/stop + warnings"] ("type of dialog (OK msg:1)")
        # "Serial logic"
        # "WAITING FORM CCYLE TO COMPLE TO PRINT QR"
        # "Wait"
        n131 = Unbundle By Name(w409) -> ("Varient number"=w408:u16, "Serial_Number"=w401:path)
        n132 = call "TAT_PLC_Data_read.vi"("Enum"=enum16{"Read", "Write"}."Read", "error in (no error)"=w402) -> ("error out"=w399:errorcluster, "Array 2"=w410:u16[])  [unwired: 8 in]
        n133 = Index Array(array=w410) -> (element #1=w412:u16, element #3=w405:u16)  [unwired: 3 in, 1 out]
        n134 = Not Equal?(x=w408, y=w412) -> (x != y?=w406:bool)
        n135 = call "Serial_Logic.vi"("error in"=w402, "Serial path"=w401) -> ("error out"=w400:errorcluster)  [unwired: 9 in]
        n136 = Equal?(x=w405, y=u16 1) -> (x = y?=w403:bool)
        n137 = Merge Errors(w399, w400) -> (w397:errorcluster)
        n138 = call <userlib>:"Boolean Trigger__ogtk.vi"("Boolean Input"=w403) -> ("Rising Edge"=w417:bool, "Falling Edge"=w415:bool)  [unwired: 1 in]
        n139 = Build Array(w417, w415, w406) -> (w416:bool[])
        n140 = Search 1D Array(1D array=w416, element=TRUE ("Boolean Input")) -> (index of element=w414:i32)  [unwired: 1 in]
        n141 = case shown="1" w414 {
          tunnel: [Ass._Loop_Control."Wait" ("Enum") Ass._Loop_Control."Start Cycle" ("Enum") Ass._Loop_Control."GENERATE_QR_PRNT" ("Enum") Ass._Loop_Control."Cluster_update" ("Enum")] -> w407
          frame -1, Default {
          }
          frame 0 {
            # "CYCYLE START BIT"
          }
          frame 1 {
            # "CYCLE END STORE RLT"
          }
          frame 2 {
            # "CLUSTER UPDATE"
          }
        }
        n142 = call <vilib>:"Simple Error Handler.vi"("type of dialog (OK msg:1)"=w398, "error in (no error)"=w397) -> ("error out"=w396:errorcluster)  [unwired: 3 in, 4 out]
      }
      frame "Start Cycle" {
        n143 = local write "CYCLE STATUS STATION 1"("Cycle started" ("Cycle Status")) -> ()
      }
      frame "GENERATE_QR_PRNT" {
        w429 = T5 1 items=["no dialog", "OK message", "continue or stop message", "OK message + warnings", "continue/stop + warnings"] ("type of dialog (OK msg:1)")
        # "VARIENT NAME REMAIN TO ADD"
        # "GENERATE QR CODE AND PRINT QR CODE"
        n144 = Unbundle By Name(w433) -> ("Station1 printer IP"=w436:string, "Part PRN path"=w441:path, "Serial_Number"=w430:path)
        n145 = call "TAT_PLC_Data_read.vi"("Enum"=enum16{"Read", "Write"}."Read", "error in (no error)"=w438) -> ("error out"=w437:errorcluster, "Array 2"=w439:u16[])  [unwired: 8 in]
        n146 = Index Array(array=w439) -> (element #5=w431:u16)  [unwired: 5 in, 4 out]
        n147 = case shown="1" w431 {
          tunnel: w441 -> [_ w470]
          tunnel: w437 -> [w445 w453]
          tunnel: w431 -> [_ _]
          tunnel: [w445 w461] -> w428
          tunnel: w436 -> [_ w459]
          tunnel: w433 -> [w442 w447]
          tunnel: [FALSE TRUE] -> w435
          tunnel: [Ass._Loop_Control."Wait" ("Enum") Ass._Loop_Control."SaveReport " ("Enum")] -> w434
          tunnel: [w442 w456] -> w432
          tunnel: w430 -> [_ w451]
          frame 0, Default {
            # "cycyle not ok"
          }
          frame 1 {
            # "Cycle OK"
            n148 = call "Serial_ini.vi"("error in"=w453, "Serial path"=w451, "Enum"=enum16{"Write", "Read"}."Read") -> ("error out"=w454:errorcluster, "Count"=w450:u32)  [unwired: 5 in, 2 out]
            n149 = Increment(x=w450) -> (x+1=w449:u32)
            n150 = Number To Decimal String(number=w449) -> (decimal integer string=w448:string)  [unwired: 1 in]
            n151 = Bundle By Name(cluster=w447, "Current Serial Number"=w448) -> (w446:T3)
            n152 = call "PRN Generation_Station1.vi"("Part PRN QR"=w470, "error in (no error)"=w454, "Cluster"=w446) -> ("QR Code"=w455:string, "PRN to Print"=w460:string, "error out"=w462:errorcluster)  [unwired: 5 in]
            n153 = TCP Open Connection(address=w459, remote port or service name=u16 6101, error in (no error)=w462) -> (connection ID=w465:refnum<k5>, error out=w466:errorcluster)  [unwired: 2 in]
            n154 = TCP Write(connection ID=w465, data in=w460, error in (no error)=w466) -> (connection ID out=w463:refnum<k5>, error out=w468:errorcluster)  [unwired: 1 in, 1 out]
            n155 = call "Stall Data Flow.vim"("value in"=w468, "milliseconds to wait"=u32 1000) -> ("value out"=w464:errorcluster)  [unwired: 1 out]
            n156 = TCP Close Connection(connection ID=w463, error in (no error)=w464) -> (error out=w461:errorcluster)  [unwired: 1 in, 1 out]
            n157 = Bundle By Name(cluster=w446, "Station1_QR"=w455) -> (w456:T3)
            n158 = local write "QR STATION 1"(w455) -> ()
          }
        }
        n159 = local write "RESULT STATION 1"(w435) -> ()
        n160 = call <vilib>:"Simple Error Handler.vi"("type of dialog (OK msg:1)"=w429, "error in (no error)"=w428) -> ("error out"=w427:errorcluster)  [unwired: 3 in, 4 out]
      }
      frame "SaveReport " {
        w474 = T5 1 items=["no dialog", "OK message", "continue or stop message", "OK message + warnings", "continue/stop + warnings"] ("type of dialog (OK msg:1)")
        (unwired) string[] ["Date", "Time", "Model_No", "Part_Name", "Part_No", "Torishi_Code", "Shift", "Cycle_Time", "Station1_Rst", "Packaging_Qty", "Serial_No", "QR_Code", "Station2_Rst"] ("columns 2")
        # "Save Barcode code AND RESULT in SQL"
        n161 = call "Station1_Data_Log.vi"("error in (no error)"=w485, "Cluster"=w480) -> ("error out"=w482:errorcluster)  [unwired: 8 in, 1 out]
        n162 = Unbundle By Name(w480) -> ("Serial_Number"=w479:path, "Current Serial Number"=w476:string)
        n163 = Decimal String To Number(string=w476, default (0L)=u32 0 ("default (0 I32)")) -> (number=w471:u32)  [unwired: 1 in, 1 out]
        "SERIAL NO.:- 2" <- w471
        n164 = call "Serial_ini.vi"("error in"=w482, "Serial path"=w479, "Enum"=enum16{"Write", "Read"}."Read") -> ("error out"=w483:errorcluster, "Shift"=w477:string, "Date"=w478:string)  [unwired: 5 in, 1 out]
        n165 = call "Serial_ini.vi"("error in"=w483, "Serial path"=w479, "Date"=w478, "Count"=w471, "Shift"=w477, "Enum"=enum16{"Write", "Read"}."Write") -> ("error out"=w473:errorcluster)  [unwired: 2 in, 3 out]
        n166 = call <vilib>:"Simple Error Handler.vi"("type of dialog (OK msg:1)"=w474, "error in (no error)"=w473) -> ("error out"=w472:errorcluster)  [unwired: 3 in, 4 out]
      }
      frame "Cycle End" {
      }
      frame "Stop" {
        n167 = local write "CYCLE STATUS STATION 1"("STATION STOP" ("Cycle Status")) -> ()
      }
    }
    n168 = global read "Global 1.vi" "PLC Communication"() -> (→"PLC STATUS:-":bool)
    n169 = call "TAT_PLC_Data_read.vi"("Enum"=enum16{"Read", "Write"}."Read") -> ("Array 2"=w111:u16[])  [unwired: 9 in, 1 out]
    n170 = Index Array(array=w111, index #1=2 ("index"), index #2=4 ("index"), index #3=6 ("index")) -> (element #1=w109:u16, element #2=w104:u16, element #3=→"CYCLE TIME:-":u16)
    n171 = case shown="0, Default" w109 {
      tunnel: [FALSE TRUE] -> w108
      frame 0, Default {
      }
      frame 1 {
      }
    }
    "CYCLE START:-" <- w108
    n172 = case shown="0, Default" w104 {
      tunnel: [FALSE TRUE] -> w84
      frame 0, Default {
      }
      frame 1 {
      }
    }
    "CYCLE RESULT:-" <- w84
    n173 = call "TAT_LABVIEW_TO_PLC.vi"("Enum"=enum16{"Read", "Write"}."Read") -> ("error out"=w101:errorcluster, "Array 2"=w100:bool[])  [unwired: 9 in]
    n174 = Replace Array Subset(array=w100, new element=TRUE ("new element/subarray"), index=0) -> (w99:bool[])
    n175 = call "TAT_LABVIEW_TO_PLC.vi"("Enum"=enum16{"Read", "Write"}."Write", "error in (no error)"=w101, "Array"=w99) -> ("error out"=w85:errorcluster)  [unwired: 7 in, 1 out]
    n176 = call "TAT_PLC_Data_read_BOLLEAN.vi"("Enum"=enum16{"Read", "Write"}."Read", "error in (no error)"=w85) -> ("Array 2"=w88:bool[])  [unwired: 8 in, 1 out]
    n177 = Index Array(array=w88) -> (element #1=→"CAP SEAL:-":bool, element #2=→"HOSE:-":bool, element #3=→"RBC-M-H:-":bool, element #4=→"RBC-M-EX:-":bool, element #5=→"PYIB-MD:-":bool, element #6=→"PYIB-MD-EX:-":bool, element #7=→"DUAL:-":bool, element #8=→"PY1B-D:-":bool, element #9=→"PY1B-D-EX:-":bool)  [unwired: 9 in]
    n178 = Select(t=Ass._Loop_Control."Stop" ("Enum"), s="Stop", f=w115) -> (s? t:f=w116:T4)
    n179 = Wait (ms)(milliseconds to wait=u32 150) -> ()  [unwired: 1 out]
    n180 = Select(t=Ass._Loop_Control."Stop" ("Enum"), s="Stop", f=w113) -> (s? t:f=w130:T4)
  }
  n181 = disable-structure shown="Disabled" {
    frame Disabled {
    }
    frame Enabled {
    }
  }
  n182 = property class="App"() -> ("App.Kind"=w38:T6)  [unwired: 2 in, 2 out]
  n183 = Merge Errors(w47, w39) -> (w45:errorcluster)
  n184 = Unbundle By Name(w11) -> ("connection reference"=w12:T1)
  n185 = call <vilib>:"Simple Error Handler.vi"("type of dialog (OK msg:1)"=w42, "error in (no error)"=w45) -> ("error out"=w14:errorcluster)  [unwired: 3 in, 4 out]
  "error out" <- w14
  n186 = call <vilib>:"Clear Errors.vi"("error in (no error)"=w14) -> ("error out"=w19:errorcluster)  [unwired: 5 in, 1 out]
  n187 = case shown="\"Run Time System\"" w38 {
    tunnel: w14 -> [_ w496]
    frame "invalid app kind", Default {
    }
    frame "Run Time System" {
      n188 = call <vilib>:"Clear Errors.vi"("error in (no error)"=w496) -> ("error out"=w495:errorcluster)  [unwired: 5 in, 1 out]
      n189 = invoke class="VI" method="FP.Close"(error in=w495) -> ()  [unwired: 2 in, 3 out]
    }
  }
  n190 = call <vilib>:"Clear Errors.vi"("error in (no error)"=w14) -> ("error out"=w13:errorcluster)  [unwired: 5 in, 1 out]
  n191 = call "TAT_LABVIEW_TO_PLC.vi"("Enum"=enum16{"Read", "Write"}."Read", "error in (no error)"=w19) -> ("error out"=w22:errorcluster, "Array 2"=w23:bool[])  [unwired: 8 in]
  n192 = call <vilib>:"DB Tools Close Connection.vi"("error in (no error)"=w13, "connection reference"=w12) -> ()  [unwired: 5 in, 1 out]
  n193 = Insert Into Array(array=w23, new element=TRUE ("new element/subarray")) -> (w24:bool[])  [unwired: 1 in]
  n194 = call "TAT_LABVIEW_TO_PLC.vi"("Enum"=enum16{"Read", "Write"}."Write", "error in (no error)"=w22, "Array"=w24) -> ()  [unwired: 7 in, 2 out]
  "CYCLE STATUS STATION 1" <- ""
  "QR STATION 1" <- ""
  "RESULT STATION 1" <- FALSE ("want seconds? (F)")
